vi "arm PID.vi"(0 "Desired Rate":dbl) -> (1 "Motor Output":dbl)   [LabVIEW 2012]
uses:
  <vilib>/addons/control/pid/pid.llb/PID (DBL).vi
  <vilib>/addons/control/pid/NI_PID_pid.lvlib
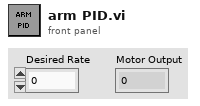
[diagram p1: front panel]
types:
  T1 = typedef "subStates.ctl" = enum16{"null", "wait", "driver control", "auto", "manual override", "hold position", "rotate", "feeder", "shoot", "end"}
  T2 = cluster{"proportional gain (Kc)":dbl, "integral time (Ti, min)":dbl, "derivative time (Td, min)":dbl}
  T3 = typedef "WPI_EncoderDevRef.ctl" = cluster{"DevStatus":errorcluster, "EncoderIndex":T4, "CounterIndex":T5, "DistancePerCount":dbl, "Decoding Type":T6}
  T4 = typedef "FPGA_EncoderIdx.ctl" = enum8{"Enc 0", "Enc 1", "Enc 2", "Enc 3", "Invalid"}
  T5 = typedef "FPGA_CounterCtrSystemIndex.ctl" = enum8{"Ctr 0", "Ctr 1", "Ctr 2", "Ctr 3", "Ctr 4", "Ctr 5", "Ctr 6", "Ctr 7", "Invalid"}
  T6 = typedef "WPI_EncoderType.ctl" = enum16{"1x", "2x", "4x"}
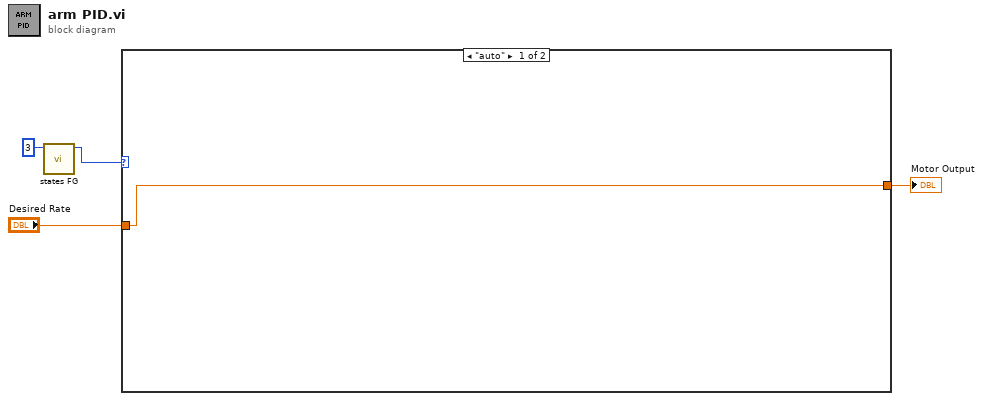
[diagram p0: block diagram]
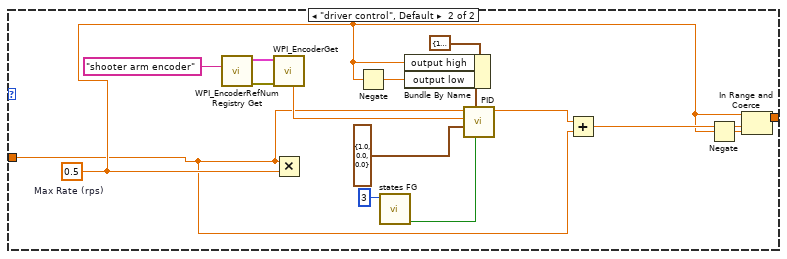
[diagram p2: hidden frame]
diagram:
  n1 = call "states FG.vi"("Loop ID"=3) -> ("subState out"=w1:T1)  [unwired: 7 in, 3 out]
  n2 = case shown="\"auto\"" w1 {
    tunnel: [w5 w12] -> w4
    tunnel: "Desired Rate" -> [w5 w6]
    frame "auto" {
    }
    frame "driver control", Default {
      w8 = 0.5  # Max Rate (rps)
      n3 = call <vilib>:"WPI_EncoderRefNum Registry Get.vi"("refnum name"="shooter arm encoder") -> ("error out"=w20:errorcluster, "EncoderDevRef"=w19:T3)  [unwired: 9 in]
      n4 = call <vilib>:"WPI_EncoderGet.vi"("error in (no error)"=w20, "EncoderDevRef"=w19) -> ("Rate"=w18:dbl)  [unwired: 4 in, 5 out]
      n5 = Multiply(x=w6, y=w8) -> ()  [unwired: 1 out]
      n6 = Negate(x=w8) -> (-x=w9:dbl)
      n7 = call "states FG.vi"("Loop ID"=3) -> ("first call?"=w15:bool)  [unwired: 7 in, 3 out]
      n8 = Bundle By Name(cluster=cluster{"output high":dbl, "output low":dbl} {"output high"=100.0, "output low"=-100.0} ("output range"), "output high"=w8, "output low"=w9) -> (w11:cluster{"output high":dbl, "output low":dbl})
      n9 = call-poly <vilib>:"PID.vi"("reinitialize? (F)"=w15, "output range"=w11, "PID gains"=T2 {"proportional gain (Kc)"=1.0, "integral time (Ti, min)"=0.0, "derivative time (Td, min)"=0.0}, "process variable"=w18, "setpoint"=w6) -> ("output"=w14:dbl)  [unwired: 5 in, 1 out]
      n10 = Add(x=w14, y=w6) -> (x+y=w13:dbl)
      n11 = Negate(x=w8) -> (-x=w7:dbl)
      n12 = In Range and Coerce(upper limit=w8, x=w13, lower limit=w7) -> (coerced(x)=w12:dbl)  [unwired: 1 out]
    }
  }
  "Motor Output" <- w4
